vi "HexStringtoNormalString.vi"(11 "String in (hex).":string) -> (3 "String out (normal)":string)   [LabVIEW 2016]
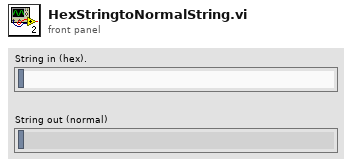
[diagram p1: front panel]
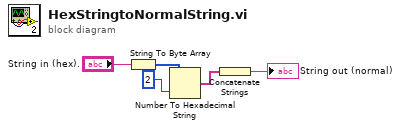
[diagram p0: block diagram]
diagram:
  n1 = String To Byte Array(string="String in (hex).") -> (unsigned byte array=w2:u8[])
  n2 = Number To Hexadecimal String(1:i16 2 ("width (-)"), 2:w2) -> (0:w4:string[])
  n3 = Concatenate Strings(w4) -> (→"String out (normal)":string)
